vi "ParseTimingInfo.vi"(5 "Input String":string="Clock1\tRG+\t-10.0\t+10.0\t2\t0\t0") -> (0 "Value":sgl format="%.1f", 1 "Name":string, 2 "Maximum":sgl format="%.2f", 3 "Minimum":sgl format="%.2f")   [LabVIEW 2014]
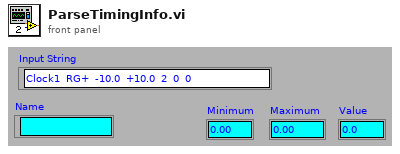
[diagram p1: front panel]
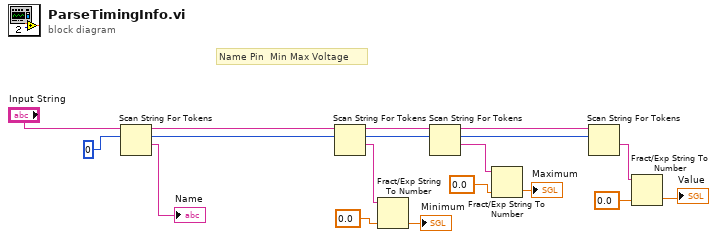
[diagram p0: block diagram]
diagram:
  # "Name Pin  Min Max Voltage"
  n1 = Scan String For Tokens(8:0 ("offset"), 9:"Input String") -> (1:→"Name":string, 2:w1:i32, 3:w2:string)  [unwired: 4 in, 1 out]
  n2 = Scan String For Tokens(8:w1, 9:w2) -> (1:w18:string, 2:w16:i32, 3:w17:string)  [unwired: 4 in, 1 out]
  n3 = Fract/Exp String To Number(string=w18, default (0 dbl)=sgl 0.0 ("default (0L)")) -> (number=→"Minimum":sgl)  [unwired: 2 in, 1 out]
  n4 = Scan String For Tokens(8:w16, 9:w17) -> (1:w15:string, 2:w5:i32, 3:w6:string)  [unwired: 4 in, 1 out]
  n5 = Fract/Exp String To Number(string=w15, default (0 dbl)=sgl 0.0 ("default (0L)")) -> (number=→"Maximum":sgl)  [unwired: 2 in, 1 out]
  n6 = Scan String For Tokens(8:w5, 9:w6) -> (1:w12:string)  [unwired: 4 in, 3 out]
  n7 = Fract/Exp String To Number(string=w12, default (0 dbl)=sgl 0.0) -> (number=→"Value":sgl)  [unwired: 2 in, 1 out]
